vi "Untitled 4.vi"   [LabVIEW 2013]
uses:
  <vilib>/Rock Robotics/Network Tables/SD Read Number.vi
types:
  T1 = typedef "WPI_JoystickButtonState.ctl" = cluster{"Button 1":bool, "Button 2":bool, "Button 3":bool, "Button 4":bool, "Button 5":bool, "Button 6":bool, "Button 7":bool, "Button 8":bool, "Button 9":bool, "Button 10":bool, "Button 11":bool, "Button 12":bool}
  T2 = cluster{"Axes":cluster{"Joystick 1":cluster{"X Axis":dbl, "Y Axis":dbl}, "Triggers":dbl, "Joystick 2":cluster{"X Axis":dbl, "Y Axis":dbl}}, "Buttons":T1}
  T3 = cluster{"Joystick 1":cluster{"X Axis":dbl, "Y Axis":dbl}, "Triggers":dbl, "Joystick 2":cluster{"X Axis":dbl, "Y Axis":dbl}}
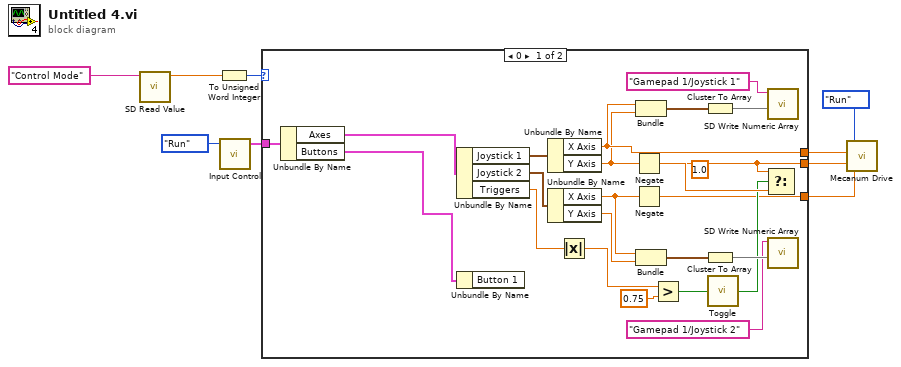
[diagram p0: block diagram]
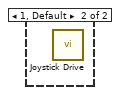
[diagram p2: hidden frame]
diagram:
  n1 = call-poly <vilib>:"SD Read Value.vi"("Name"="Control Mode") -> ("Numeric"=w8:dbl)  [unwired: 8 in, 2 out]
  n2 = To Unsigned Word Integer(number=w8) -> (unsigned 16bit integer=w7:u16)
  n3 = call "Input Control.vi"("State"=enum16{"Open", "Run", "End"}."Run") -> ("Gamepad"=w5:T2)  [unwired: 2 in, 2 out]
  n4 = case shown="0" w7 {
    tunnel: w5 -> [w31 _]
    tunnel: [w12 _] -> w3
    tunnel: [w11 _] -> w2
    tunnel: [w10 _] -> w1
    frame 0 {
      (unwired) 1.0 ("Division")
      n5 = Unbundle By Name(w31) -> ("Axes"=w14:T3, "Buttons"=w13:T1)
      n6 = Unbundle By Name(w14) -> ("Joystick 1"=w30:cluster{"X Axis":dbl, "Y Axis":dbl}, "Joystick 2"=w22:cluster{"X Axis":dbl, "Y Axis":dbl}, "Triggers"=w19:dbl)
      n7 = Unbundle By Name(w13) -> ()  [unwired: 1 out]
      n8 = Unbundle By Name(w30) -> ("X Axis"=w12:dbl, "Y Axis"=w11:dbl)
      n9 = Unbundle By Name(w22) -> ("X Axis"=w23:dbl, "Y Axis"=w25:dbl)
      n10 = Absolute Value(x=w19) -> (abs(x)=w18:dbl)
      n11 = Negate(x=w11) -> (-x=w20:dbl)
      n12 = Negate(x=w23) -> (-x=w10:dbl)
      n13 = Bundle("X Axis"=w12, "Y Axis"=w11) -> (w21:cluster{"X Axis":dbl, "Y Axis":dbl})  [unwired: 1 in]
      n14 = Bundle("X Axis"=w23, "Y Axis"=w25) -> (w27:cluster{"X Axis":dbl, "Y Axis":dbl})  [unwired: 1 in]
      n15 = Greater?(x=w18, y=0.75) -> (0:w16:bool)
      n16 = Cluster To Array(cluster=w21) -> (array=w29:dbl[])
      n17 = Cluster To Array(cluster=w27) -> (array=w26:dbl[])
      n18 = call "Toggle.vi"("Input"=w16) -> ("Latched"=w15:bool)
      n19 = Select(t=w11, s=w15, f=w20) -> ()  [unwired: 1 out]
      n20 = call <vilib>:"SD Write Numeric Array.vi"("Numeric Array"=w29, "Name"="Gamepad 1/Joystick 1") -> ()  [unwired: 8 in, 2 out]
      n21 = call <vilib>:"SD Write Numeric Array.vi"("Numeric Array"=w26, "Name"="Gamepad 1/Joystick 2") -> ()  [unwired: 8 in, 2 out]
    }
    frame 1, Default {
      n22 = call "Joystick Drive.vi"() -> ()  [unwired: 1 in]
    }
  }
  n23 = call "Mecanum Drive.vi"("Turn"=w1, "Forward/Backward"=w2, "Strafe"=w3, "State Control"=enum16{"Open", "Run", "End"}."Run") -> ()  [unwired: 4 in]
